vi "P6.vi"() -> ()   [LabVIEW 2018]
panel:
  in  "error in":errorcluster
  out "2D Picture":picture
  out "error out":errorcluster
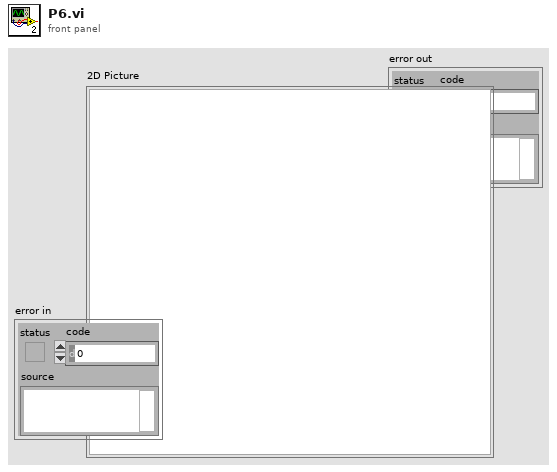
[diagram p1: front panel]
types:
  T1 = typedef "imagedata.ctl" = cluster{"image type":i32, "image depth":i32, "image":u8[], "mask":u8[], "colors":u32[], "Rectangle":cluster{"left":i16, "top":i16, "right":i16, "bottom":i16}}
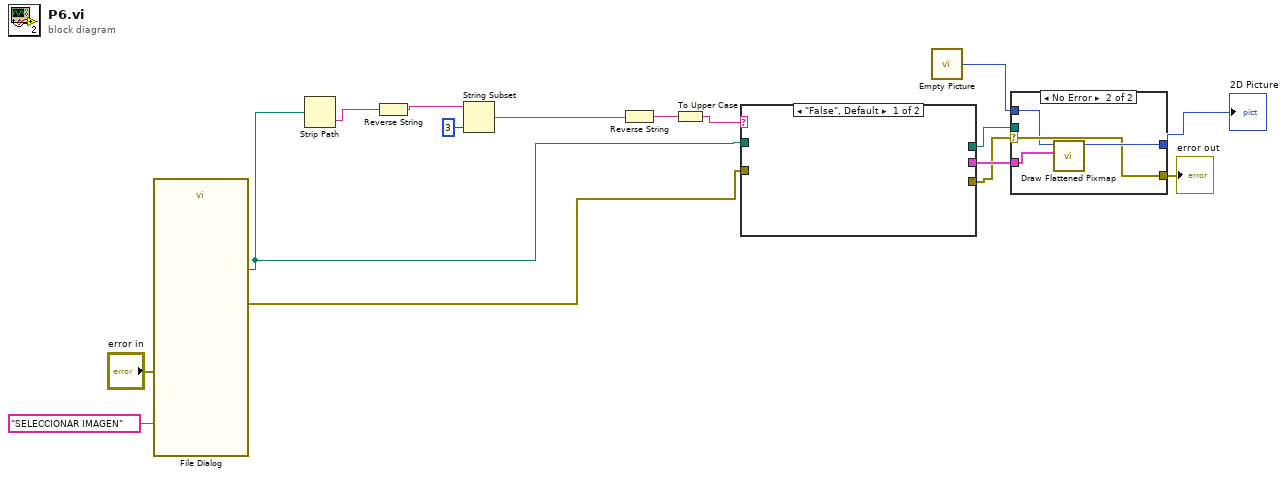
[diagram p0: block diagram]
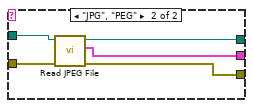
[diagram p3: hidden frame]
diagram:
  n1 = call "File Dialog"("prompt"="SELECCIONAR IMAGEN", "error in"="error in") -> ("selected path"=w9:path, "error out"=w10:errorcluster)  [unwired: 10 in, 2 out]
  n2 = Strip Path(path=w9) -> (name=w15:string)  [unwired: 1 out]
  n3 = Reverse String(1:w15) -> (0:w14:string)
  n4 = String Subset(string=w14, length (rest)=3 ("length (rest)")) -> (substring=w12:string)  [unwired: 1 in]
  n5 = Reverse String(1:w12) -> (0:w11:string)
  n6 = To Upper Case(1:w11) -> (0:w3:string)
  n7 = case shown="\"False\", Default" w3 {
    tunnel: [_ w21] -> w7
    tunnel: [_ w20] -> w8
    tunnel: [_ w19] -> w2
    tunnel: w10 -> [_ w18]
    tunnel: w9 -> [_ w17]
    frame "False", Default {
    }
    frame "JPG", "PEG" {
      n8 = call <vilib>:"Read JPEG File.vi"("error in (no error)"=w18, "path to JPEG file"=w17) -> ("error out"=w19:errorcluster, "image data"=w20:T1, "path"=w21:path)  [unwired: 7 in]
    }
  }
  n9 = call "Empty Picture"() -> ("empty picture"=w6:picture)
  n10 = case shown="No Error" w2 {
    selector: w2 -> [w23 w25]
    tunnel: w8 -> [_ w27]
    tunnel: w7 -> [_ _]
    tunnel: w6 -> [w22 w24]
    tunnel: [w23 w25] -> w5
    tunnel: [w22 w26] -> w4
    frame Error {
    }
    frame No Error {
      n11 = call <vilib>:"Draw Flattened Pixmap.vi"("image data"=w27, "picture"=w24) -> ("new picture"=w26:picture)  [unwired: 7 in]
    }
  }
  "error out" <- w5
  "2D Picture" <- w4
